vi "SetMappingsFromCustomDevice.vi"(7 "Add? (T)":bool=TRUE, 8 "error in (no error)":errorcluster, 9 "Node Path":string, 10 "GUID":string, 11 "Node Ptr":u64) -> (0 "error out":errorcluster, 3 "Section Ref out":T1 format="%.0x")   [LabVIEW 2021, in "LIN Frame Protection Addon System Explorer.lvlib"]
uses:
  LIN Frame Protection Addon System Explorer.lvlib
  <vilib>/NI VeriStand/Custom Device API/Custom Device Item Ref.ctl
  <vilib>/NI VeriStand/Custom Device Tools/Custom Device Utility Library/NI VeriStand - Search for Item by GUID.vi
  NationalInstruments.VeriStand
  NationalInstruments.VeriStand.SystemStorage
  <vilib>/NI VeriStand/Custom Device Tools/Custom Device Utility Library/Custom Device Utility Library.lvlib
  <vilib>/NI VeriStand/Custom Device API/Custom Device API.lvlib
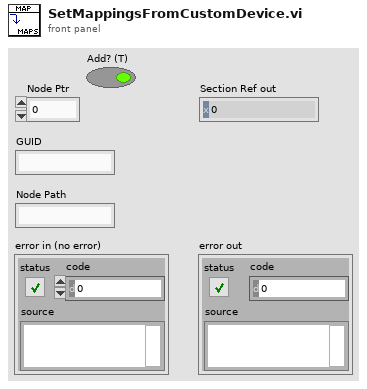
[diagram p1: front panel]
types:
  T1 = typedef "Custom Device API.lvlib/Custom Device Item Ref.ctl" = u64
  T2 = typedef "Custom Device API.lvlib/Custom Device Pointer.ctl" = refnum<k24>
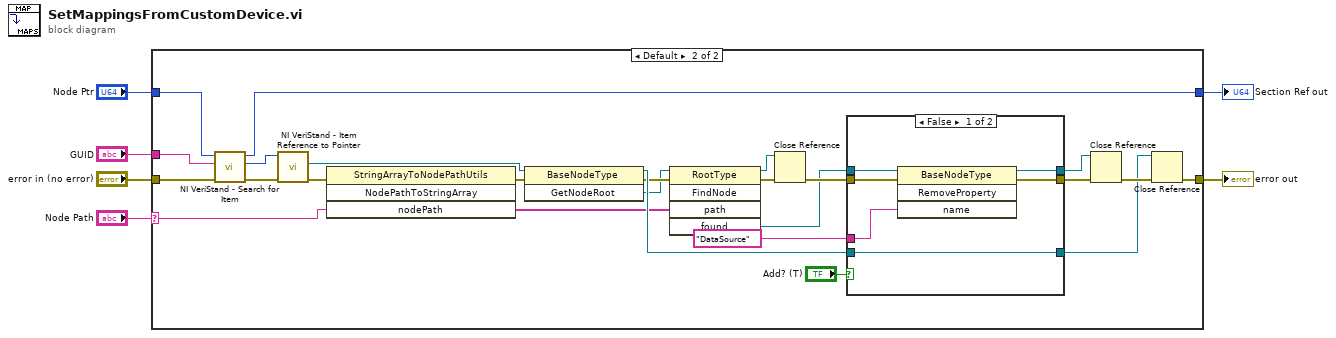
[diagram p0: block diagram]
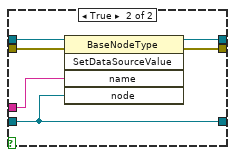
[diagram p3: hidden frame]
diagram:
  n1 = case shown="Default" "Node Path" {
    selector: "Node Path" -> [_ w9]
    tunnel: [w7 w27] -> w6
    tunnel: [w8 w19] -> w5
    tunnel: "error in (no error)" -> [w7 w18]
    tunnel: "GUID" -> [_ w15]
    tunnel: "Node Ptr" -> [w8 w14]
    frame "" {
    }
    frame Default {
      n2 = call-poly <vilib>:"NI VeriStand - Search for Item.vi"("error in"=w18, "Item GUID"=w15, "Section Ref in"=w14) -> ("error out"=w17:errorcluster, "Item Ref"=w16:T1, "Section Ref out"=w19:T1)  [unwired: 5 in, 1 out]
      n3 = call <vilib>:"NI VeriStand - Item Reference to Pointer.vi"("error in (no error)"=w17, "Item Ref in"=w16) -> ("error out"=w21:errorcluster, "Node Pointer"=w22:T2)  [unwired: 6 in, 2 out]
      n4 = invoke class="StringArrayToNodePathUtils" method="NodePathToStringArray"(error in=w21, "nodePath"=w9) -> (error out=w24:errorcluster, "NodePathToStringArray"=w20:string[])  [unwired: 2 in, 2 out]
      n5 = invoke class="BaseNodeType" method="GetNodeRoot"(reference=w22, error in=w24) -> (reference out=w28:T2, error out=w25:errorcluster, "GetNodeRoot"=w23:refnum<k24>)  [unwired: 1 in]
      n6 = invoke class="RootType" method="FindNode"(reference=w23, error in=w25, "path"=w20) -> (reference out=w33:refnum<k24>, error out=w32:errorcluster, "found"=w12:refnum<k24>)  [unwired: 2 in, 2 out]
      n7 = Close Reference(reference=w33, error in (no error)=w32) -> (error out=w13:errorcluster)
      n8 = case shown="False" "Add? (T)" {
        tunnel: [w36 w45] -> w31
        tunnel: [w37 w44] -> w29
        tunnel: w28 -> [w34 w40]
        tunnel: w13 -> [w38 w43]
        tunnel: w12 -> [w39 w42]
        tunnel: "DataSource" ("name") -> [w35 w41]
        tunnel: [w34 w40] -> w10
        frame False {
          n9 = invoke class="BaseNodeType" method="RemoveProperty"(reference=w39, error in=w38, "name"=w35) -> (reference out=w36:refnum<k24>, error out=w37:errorcluster)  [unwired: 1 in, 2 out]
        }
        frame True {
          n10 = invoke class="BaseNodeType" method="SetDataSourceValue"(reference=w42, error in=w43, "name"=w41, "node"=w40) -> (reference out=w45:refnum<k24>, error out=w44:errorcluster)  [unwired: 1 in, 3 out]
        }
      }
      n11 = Close Reference(reference=w31, error in (no error)=w29) -> (error out=w30:errorcluster)
      n12 = Close Reference(reference=w10, error in (no error)=w30) -> (error out=w27:errorcluster)
    }
  }
  "error out" <- w6
  "Section Ref out" <- w5
